vi "PH_TKTDS-30xx.get physical Channel Name.vi"(0 "i ref in":refnum<vi>, 2 "GUI Element Name":string, 5 "error in":errorcluster) -> (14 "i ref out":refnum<vi>, 17 "Physical Channel Name":string, 18 "Waveform Limits":T1={"Start"=1, "End"=10000}, 19 "error out":errorcluster)   [LabVIEW 2014, in "PH_TKTDS-30xx.lvlib"]
doc: "This VI queries the physical channel name, defined by the GUI element name."
uses:
  PH_TKTDS-30xx.lvlib
  PH_TKTDS-30xx.Waveform Limits.ctl
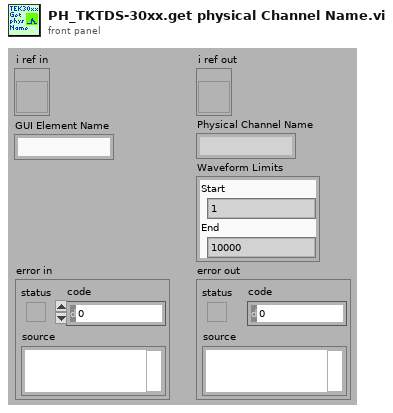
[diagram p1: front panel]
types:
  T1 = typedef "PH_TKTDS-30xx.lvlib/PH_TKTDS-30xx.Waveform Limits.ctl" = cluster{"Start":i32, "End":i32}
  T2 = typedef "PH_TKTDS-30xx.lvlib/PH_TKTDS-30xx.i attribute.ctl" = cluster{"Default VISA Resource":string, "VISA Resource Name":refnum<visa-resource-name>, "Revision":cluster{"Instrument Driver":string, "Instrument Firmware":string}, "Selftest":cluster{"Result":u32, "Message":string}, "Channels":T3[], "Trigger Configuration":T4, "Acquisition Configuration":T5, "Fetched Waveforms":T6[], "GUI Refs":T7, "State":T8, "Error Message":string, "Allow Prdc Loop?":bool}
  T3 = typedef "PH_TKTDS-30xx.lvlib/PH_TKTDS-30xx.Channel Config.ctl" = cluster{"Channel Name":string, "Input Impedance":string, "Max Input Frequency":string, "Vertical Coupling":i32, "Channel Enabled":bool, "Probe Attenuation":dbl, "Vertical Range":dbl, "Vertical Offset":dbl, "Waveform Limits":T1}
  T4 = typedef "PH_TKTDS-30xx.lvlib/PH_TKTDS-30xx.Trigger Config.ctl" = cluster{"Source":string, "Slope":i32, "Level [V]":dbl}
  T5 = typedef "PH_TKTDS-30xx.lvlib/PH_TKTDS-30xx.Acquisition Config.ctl" = cluster{"Time base":dbl, "Record Length":u16, "Start Time":dbl, "Type":i32, "Continuous":bool}
  T6 = typedef "PH_TKTDS-30xx.lvlib/PH_TKTDS-30xx.fetched Waveform.ctl" = cluster{"Source":string, "Actual Points":u32, "Initial X":dbl, "X Increment":dbl, "Waveform Array":dbl[]}
  T7 = typedef "PH_TKTDS-30xx.lvlib/PH_TKTDS-30xx.GUI Refs.ctl" = cluster{"Trigger":refnum<vi>, "Acquisition":refnum<vi>, "State":refnum<vi>, "Delete":refnum<vi>, "Channel to be positioned":refnum<vi>, "Postion":refnum<vi>, "Display Intensity":refnum<vi>, "VISA Resource":refnum<vi>, "Channels":refnum<vi>[], "Graphs":refnum<vi>[]}
  T8 = typedef "PH_StatusHandler.lvlib/PH_StatusHandler.Status.ctl" = i16
  T9 = typedef "PH_TKTDS-30xx.Waveform Limits.ctl" = cluster{"Start":i32, "End":i32}
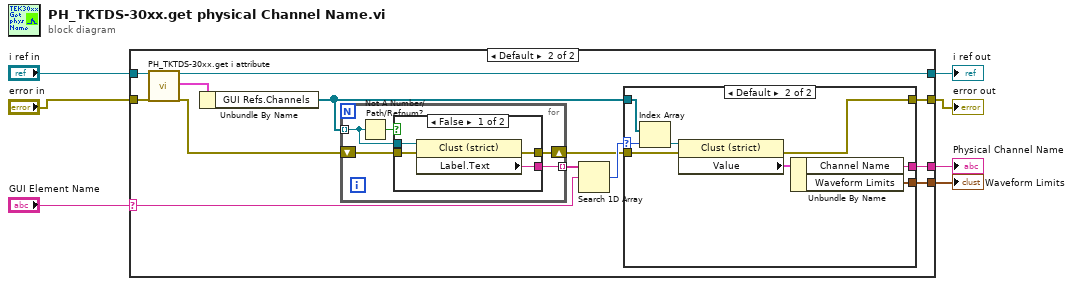
[diagram p0: block diagram]
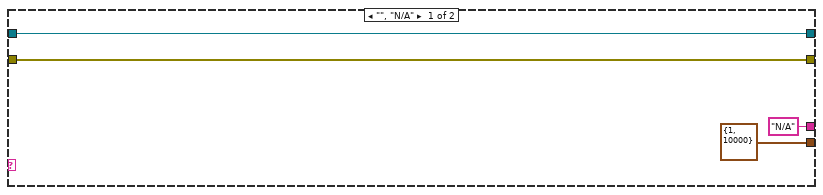
[diagram p2: hidden frame]
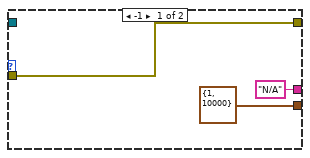
[diagram p3: hidden frame]
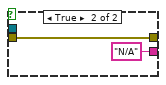
[diagram p4: hidden frame]
diagram:
  n1 = case shown="Default" "GUI Element Name" {
    selector: "GUI Element Name" -> [_ w13]
    tunnel: [w11 w23] -> w7
    tunnel: [w10 w17] -> w6
    tunnel: "error in" -> [w10 w16]
    tunnel: "i ref in" -> [w11 w15]
    tunnel: ["N/A" ("Channel Name") w14] -> w3
    tunnel: [T1 {"Start"=1, "End"=10000} ("Waveform Limits") w12] -> w1
    frame "", "N/A" {
    }
    frame Default {
      n2 = call "PH_TKTDS-30xx.get i attribute.vi"("i ref in"=w15, "error in (no error)"=w16) -> ("i ref out"=w23:refnum<vi>, "i attribute"=w24:T2, "error out"=w21:errorcluster)  [unwired: 15 in]
      n3 = Unbundle By Name(w24) -> ("GUI Refs.Channels"=w20:refnum<vi>[])
      n4 = for {
        tunnel: w20 -> [w37] mode=indexing
        shift-right: [w40] -> w18
        shift-left: w21 -> [w39]
        tunnel: [w36] -> w22 mode=indexing
        n5 = Not A Number/Path/Refnum?(number/path/refnum=w37) -> (NaN/Path/Refnum?=w38:bool)
        n6 = case shown="False" w38 {
          tunnel: w37 -> [w44 _]
          tunnel: [w43 w46] -> w40
          tunnel: w39 -> [w42 w46]
          tunnel: [w41 "N/A" ("Label.Text")] -> w36
          frame False {
            n7 = property class="Clust (strict)"(reference=w44, error in=w42) -> (error out=w43:errorcluster, "Label.Text"=w41:string)  [unwired: 1 out]
          }
          frame True {
          }
        }
      }
      n8 = Search 1D Array(1D array=w22, element=w13) -> (index of element=w19:i32)  [unwired: 1 in]
      n9 = case shown="Default" w19 {
        selector: w19 -> [_ w31]
        tunnel: w20 -> [_ w35]
        tunnel: w18 -> [w27 w33]
        tunnel: [w27 w32] -> w17
        tunnel: ["N/A" ("Channel Name") w29] -> w14
        tunnel: [T1 {"Start"=1, "End"=10000} ("Waveform Limits") w28] -> w12
        frame -1 {
        }
        frame Default {
          n10 = Index Array(array=w35, index=w31) -> (element=w34:refnum<vi>)
          n11 = property class="Clust (strict)"(reference=w34, error in=w33) -> (error out=w32:errorcluster, "Value"=w30:T3)  [unwired: 1 out]
          n12 = Unbundle By Name(w30) -> ("Channel Name"=w29:string, "Waveform Limits"=w28:T9)
        }
      }
    }
  }
  "error out" <- w6
  "i ref out" <- w7
  "Physical Channel Name" <- w3
  "Waveform Limits" <- w1
